vi "nanocal -- nuclear schottky fit -- 2x2 -- V9.vi"() -> ()   [LabVIEW 2021] (continued)
\"Imoff\" -> 0.000000000000   ,  \"στ1\" -> 0.008245172960   ,  \"στS\" -> 0.001836119711   ,  \"στN\" -> 0.000000000000    |>   , \n\"IDS0301_210831_RAW_cal__sam_\" ->   <|    \"ζ\" -> 0.050368719514   ,  \"τ1\" -> 0.024372679774   ,  \"τS\" -> 0.056652990002   ,  \"τN\" -> 0.018868210601   ,  \"τC\" -> 0.002169557672   ,  \"κ0\" -> 0.000000001890   ,  \"mm1\" -> 0.000100537132   ,  \"mm2\" -> 0.016885854065   ,  \"mm3\" -> 0.088880953022   ,  \"T\" -> 0.300000000000   ,  \"B\" -> 12.000000000000   ,  \"θ\" -> 30.000000000000   ,  \"Reoff\" -> -5240963.855421677230   ,  \"Imoff\" -> 0.000000000000   ,  \"στ1\" -> 0.000000000000   ,  \"στS\" -> 0.000000000000   ,  \"στN\" -> 0.000000000000    |>   , \n\"IDS0302_210831_RAW_cal__ref_\" ->   <|    \"ζ\" -> 0.118276511674   ,  \"τ1\" -> 0.024667236768   ,  \"τS\" -> 0.048709348590   ,  \"τN\" -> 0.031529020299   ,  \"τC\" -> 0.001279390112   ,  \"κ0\" -> 0.000000001362   ,  \"mm1\" -> 0.000132517053   ,  \"mm2\" -> 0.013437351030   ,  \"mm3\" -> 0.102105442061   ,  \"T\" -> 0.250000000000   ,  \"B\" -> 12.000000000000   ,  \"θ\" -> 30.000000000000   ,  \"Reoff\" -> -14030120.481927707800   ,  \"Imoff\" -> 0.000000000000   ,  \"στ1\" -> 0.005527591080   ,  \"στS\" -> 0.002366766012   ,  \"στN\" -> 0.000000000000    |>   , \n\"IDS0302_210831_RAW_cal__sam_\" ->   <|    \"ζ\" -> 0.070275268573   ,  \"τ1\" -> 0.028026457127   ,  \"τS\" -> 0.065297867120   ,  \"τN\" -> 0.040008645873   ,  \"τC\" -> 0.001817885465   ,  \"κ0\" -> 0.000000001504   ,  \"mm1\" -> 0.000116520135   ,  \"mm2\" -> 0.015851021970   ,  \"mm3\" -> 0.126583756963   ,  \"T\" -> 0.250000000000   ,  \"B\" -> 12.000000000000   ,  \"θ\" -> 30.000000000000   ,  \"Reoff\" -> -8554216.867469877010   ,  \"Imoff\" -> 0.000000000000   ,  \"στ1\" -> 0.000000000000   ,  \"στS\" -> 0.000000000000   ,  \"στN\" -> 0.000000000000    |>   , \n\"IDS0303_210831_RAW_cal__ref_\" ->   <|    \"ζ\" -> 0.210201005272   ,  \"τ1\" -> 0.036306230706   ,  \"τS\" -> 0.066320996268   ,  \"τN\" -> 0.080911010033   ,  \"τC\" -> 0.001077377701   ,  \"κ0\" -> 0.000000001046   ,  \"mm1\" -> 0.000185060428   ,  \"mm2\" -> 0.014681839337   ,  \"mm3\" -> 0.200697030676   ,  \"T\" -> 0.200000000000   ,  \"B\" -> 12.000000000000   ,  \"θ\" -> 30.000000000000   ,  \"Reoff\" -> -29165662.650602400300   ,  \"Imoff\" -> 0.000000000000   ,  \"στ1\" -> 0.007631270383   ,  \"στS\" -> 0.005042040043   ,  \"στN\" -> 0.000000000000    |>   , \n\"IDS0303_210831_RAW_cal__sam_\" ->   <|    \"ζ\" -> 0.127771364483   ,  \"τ1\" -> 0.034431916362   ,  \"τS\" -> 0.086066228156   ,  \"τN\" -> 0.103317216156   ,  \"τC\" -> 0.001469970272   ,  \"κ0\" -> 0.000000001169   ,  \"mm1\" -> 0.000164317810   ,  \"mm2\" -> 0.014420189715   ,  \"mm3\" -> 0.234898604511   ,  \"T\" -> 0.200000000000   ,  \"B\" -> 12.000000000000   ,  \"θ\" -> 30.000000000000   ,  \"Reoff\" -> -17831325.301204815500   ,  \"Imoff\" -> 0.000000000000   ,  \"στ1\" -> 0.000000000000   ,  \"στS\" -> 0.000000000000   ,  \"στN\" -> 0.000000000000    |>   , \n\"IDS0304_210831_RAW_cal__ref_\" ->   <|    \"ζ\" -> 0.269991588498   ,  \"τ1\" -> 0.042008612133   ,  \"τS\" -> 0.092789631538   ,  \"τN\" -> 0.170188261604   ,  \"τC\" -> 0.001076825929   ,  \"κ0\" -> 0.000000000745   ,  \"mm1\" -> 0.000227270912   ,  \"mm2\" -> 0.013732742400   ,  \"mm3\" -> 0.363105137001   ,  \"T\" -> 0.170000000000   ,  \"B\" -> 12.000000000000   ,  \"θ\" -> 30.000000000000   ,  \"Reoff\" -> -52171686.746987946300   ,  \"Imoff\" -> 0.000000000000   ,  \"στ1\" -> 0.010619336598   ,  \"στS\" -> 0.010896322396   ,  \"στN\" -> 0.000000000000    |>   , \n\"IDS0304_210831_RAW_cal__sam_\" ->   <|    \"ζ\" -> 0.166070461716   ,  \"τ1\" -> 0.041003941798   ,  \"τS\" -> 0.114733330952   ,  \"τN\" -> 0.164402286708   ,  \"τC\" -> 0.001371627013   ,  \"κ0\" -> 0.000000000890   ,  \"mm1\" -> 0.000193629021   ,  \"mm2\" -> 0.015725118152   ,  \"mm3\" -> 0.351948620204   ,  \"T\" -> 0.170000000000   ,  \"B\" -> 12.000000000000   ,  \"θ\" -> 30.000000000000   ,  \"Reoff\" -> -32409638.554216861700   ,  \"Imoff\" -> 0.000000000000   ,  \"στ1\" -> 0.000000000000   ,  \"στS\" -> 0.000000000000   ,  \"στN\" -> 0.000000000000    |>   , \n\"IDS0305_210831_RAW_cal__ref_\" ->   <|    \"ζ\" -> 0.281505704242   ,  \"τ1\" -> 0.044410384222   ,  \"τS\" -> 0.104666316175   ,  \"τN\" -> 0.238180601074   ,  \"τC\" -> 0.001077670144   ,  \"κ0\" -> 0.000000000630   ,  \"mm1\" -> 0.000235234007   ,  \"mm2\" -> 0.012702965231   ,  \"mm3\" -> 0.471910135265   ,  \"T\" -> 0.160000000000   ,  \"B\" -> 12.000000000000   ,  \"θ\" -> 30.000000000000   ,  \"Reoff\" -> -64885542.168674700000   ,  \"Imoff\" -> 0.000000000000   ,  \"στ1\" -> 0.013415612751   ,  \"στS\" -> 0.014884617591   ,  \"στN\" -> 0.000000000000    |>   , \n\"IDS0305_210831_RAW_cal__sam_\" ->   <|    \"ζ\" -> 0.168984978681   ,  \"τ1\" -> 0.042944879888   ,  \"τS\" -> 0.137797235983   ,  \"τN\" -> 0.201278537585   ,  \"τC\" -> 0.001423239236   ,  \"κ0\" -> 0.000000000771   ,  \"mm1\" -> 0.000204183123   ,  \"mm2\" -> 0.016435652766   ,  \"mm3\" -> 0.424102769171   ,  \"T\" -> 0.160000000000   ,  \"B\" -> 12.000000000000   ,  \"θ\" -> 30.000000000000   ,  \"Reoff\" -> -36385542.168674692500   ,  \"Imoff\" -> 0.000000000000   ,  \"στ1\" -> 0.000000000000   ,  \"στS\" -> 0.000000000000   ,  \"στN\" -> 0.000000000000    |>   , \n\"IDS0306_210831_RAW_cal__ref_\" ->   <|    \"ζ\" -> 0.013593052641   ,  \"τ1\" -> 0.010989385662   ,  \"τS\" -> 0.007947176041   ,  \"τN\" -> 0.000037757079   ,  \"τC\" -> 0.003572854733   ,  \"κ0\" -> 0.000000023548   ,  \"mm1\" -> 0.000033287498   ,  \"mm2\" -> 0.010587625602   ,  \"mm3\" -> 0.012034800032   ,  \"T\" -> 3.100000000000   ,  \"B\" -> 12.000000000000   ,  \"θ\" -> 30.000000000000   ,  \"Reoff\" -> 0.000000000000   ,  \"Imoff\" -> 0.000000000000   ,  \"στ1\" -> 0.000000000000   ,  \"στS\" -> 0.000000000000   ,  \"στN\" -> 0.000000000000    |>   , \n\"IDS0306_210831_RAW_cal__sam_\" ->   <|    \"ζ\" -> 0.007685785961   ,  \"τ1\" -> 0.018036205476   ,  \"τS\" -> 0.008821186550   ,  \"τN\" -> 0.000090733660   ,  \"τC\" -> 0.005794291982   ,  \"κ0\" -> 0.000000024405   ,  \"mm1\" -> 0.000026803010   ,  \"mm2\" -> 0.014306219949   ,  \"mm3\" -> 0.018477889820   ,  \"T\" -> 3.100000000000   ,  \"B\" -> 12.000000000000   ,  \"θ\" -> 30.000000000000   ,  \"Reoff\" -> -62000.000000000000   ,  \"Imoff\" -> 0.000000000000   ,  \"στ1\" -> 0.000000000000   ,  \"στS\" -> 0.000000000000   ,  \"στN\" -> 0.000000000000    |>   , \n\"IDS0310_210901_RAW_cal__ref_\" ->   <|    \"ζ\" -> 0.294196069585   ,  \"τ1\" -> 0.054258754823   ,  \"τS\" -> 0.066187792705   ,  \"τN\" -> 0.210307390595   ,  \"τC\" -> 0.001028009628   ,  \"κ0\" -> 0.000000000624   ,  \"mm1\" -> 0.000231504342   ,  \"mm2\" -> 0.011693954387   ,  \"mm3\" -> 0.401200285208   ,  \"T\" -> 0.157000000000   ,  \"B\" -> 12.000000000000   ,  \"θ\" -> 45.000000000000   ,  \"Reoff\" -> -66590361.445783138300   ,  \"Imoff\" -> 0.000000000000   ,  \"στ1\" -> 0.021984252892   ,  \"στS\" -> 0.027799498625   ,  \"στN\" -> 0.000000000000    |>   , \n\"IDS0310_210901_RAW_cal__sam_\" ->   <|    \"ζ\" -> 0.295520923520   ,  \"τ1\" -> 0.054772440405   ,  \"τS\" -> 0.071814005451   ,  \"τN\" -> 0.249593767169   ,  \"τC\" -> 0.001103632155   ,  \"κ0\" -> 0.000000000625   ,  \"mm1\" -> 0.000249422174   ,  \"mm2\" -> 0.011160480416   ,  \"mm3\" -> 0.460856664381   ,  \"T\" -> 0.157000000000   ,  \"B\" -> 12.000000000000   ,  \"θ\" -> 45.000000000000   ,  \"Reoff\" -> 0.000000000000   ,  \"Imoff\" -> 0.000000000000   ,  \"στ1\" -> 0.000000000000   ,  \"στS\" -> 0.000000000000   ,  \"στN\" -> 0.000000000000    |>   , \n\"IDS0311_210901_RAW_cal__ref_\" ->   <|    \"ζ\" -> 0.508858563878   ,  \"τ1\" -> 0.072484057695   ,  \"τS\" -> 0.091005153910   ,  \"τN\" -> 0.493200178379   ,  \"τC\" -> 0.000985068264   ,  \"κ0\" -> 0.000000000428   ,  \"mm1\" -> 0.000330595844   ,  \"mm2\" -> 0.010594734788   ,  \"mm3\" -> 0.944027014014   ,  \"T\" -> 0.120000000000   ,  \"B\" -> 12.000000000000   ,  \"θ\" -> 45.000000000000   ,  \"Reoff\" -> -111015060.240963846000   ,  \"Imoff\" -> 0.000000000000   ,  \"στ1\" -> 0.030760368517   ,  \"στS\" -> 0.002434782882   ,  \"στN\" -> 0.000000000000    |>   , \n\"IDS0311_210901_RAW_cal__sam_\" ->   <|    \"ζ\" -> 0.523545279740   ,  \"τ1\" -> 0.065613539167   ,  \"τS\" -> 0.100000000000   ,  \"τN\" -> 0.424083114177   ,  \"τC\" -> 0.000911255863   ,  \"κ0\" -> 0.000000000418   ,  \"mm1\" -> 0.000311888140   ,  \"mm2\" -> 0.011767552098   ,  \"mm3\" -> 0.852909709588   ,  \"T\" -> 0.120000000000   ,  \"B\" -> 12.000000000000   ,  \"θ\" -> 45.000000000000   ,  \"Reoff\" -> 0.000000000000   ,  \"Imoff\" -> 0.000000000000   ,  \"στ1\" -> 0.000000000000   ,  \"στS\" -> 0.000000000000   ,  \"στN\" -> 0.000000000000    |>   , \n\"IDS0312_210901_RAW_cal__ref_\" ->   <|    \"ζ\" -> 0.259527657087   ,  \"τ1\" -> 0.050950801212   ,  \"τS\" -> 0.056257064354   ,  \"τN\" -> 0.162412214705   ,  \"τC\" -> 0.001029454962   ,  \"κ0\" -> 0.000000000750   ,  \"mm1\" -> 0.000209665786   ,  \"mm2\" -> 0.011572567257   ,  \"mm3\" -> 0.315618027862   ,  \"T\" -> 0.170000000000   ,  \"B\" -> 12.000000000000   ,  \"θ\" -> 45.000000000000   ,  \"Reoff\" -> -47551204.819277107700   ,  \"Imoff\" -> 0.000000000000   ,  \"στ1\" -> 0.007568346917   ,  \"στS\" -> 0.006727038440   ,  \"στN\" -> 0.000000000000    |>   , \n\"IDS0312_210901_RAW_cal__sam_\" ->   <|    \"ζ\" -> 0.273742116471   ,  \"τ1\" -> 0.052262909995   ,  \"τS\" -> 0.060554036646   ,  \"τN\" -> 0.154269705680   ,  \"τC\" -> 0.001074144337   ,  \"κ0\" -> 0.000000000753   ,  \"mm1\" -> 0.000228314156   ,  \"mm2\" -> 0.012990527394   ,  \"mm3\" -> 0.313748261000   ,  \"T\" -> 0.170000000000   ,  \"B\" -> 12.000000000000   ,  \"θ\" -> 45.000000000000   ,  \"Reoff\" -> 0.000000000000   ,  \"Imoff\" -> 0.000000000000   ,  \"στ1\" -> 0.000000000000   ,  \"στS\" -> 0.000000000000   ,  \"στN\" -> 0.000000000000    |>   , \n\"IDS0313_210901_RAW_cal__ref_\" ->   <|    \"ζ\" -> 0.214632480491   ,  \"τ1\" -> 0.045379665546   ,  \"τS\" -> 0.046142273352   ,  \"τN\" -> 0.090406420650   ,  \"τC\" -> 0.001068824468   ,  \"κ0\" -> 0.000000001040   ,  \"mm1\" -> 0.000185914799   ,  \"mm2\" -> 0.012974151189   ,  \"mm3\" -> 0.199144902930   ,  \"T\" -> 0.200000000000   ,  \"B\" -> 12.000000000000   ,  \"θ\" -> 45.000000000000   ,  \"Reoff\" -> -30325301.204819276900   ,  \"Imoff\" -> 0.000000000000   ,  \"στ1\" -> 0.006255922124   ,  \"στS\" -> 0.003795789504   ,  \"στN\" -> 0.000000000000    |>   , \n\"IDS0313_210901_RAW_cal__sam_\" ->   <|    \"ζ\" -> 0.215688135788   ,  \"τ1\" -> 0.043710888546   ,  \"τS\" -> 0.044756474141   ,  \"τN\" -> 0.090222547904   ,  \"τC\" -> 0.001049781785   ,  \"κ0\" -> 0.000000001047   ,  \"mm1\" -> 0.000183308759   ,  \"mm2\" -> 0.012306282012   ,  \"mm3\" -> 0.196363475241   ,  \"T\" -> 0.200000000000   ,  \"B\" -> 12.000000000000   ,  \"θ\" -> 45.000000000000   ,  \"Reoff\" -> 0.000000000000   ,  \"Imoff\" -> 0.000000000000   ,  \"στ1\" -> 0.000000000000   ,  \"στS\" -> 0.000000000000   ,  \"στN\" -> 0.000000000000    |>   , \n\"IDS0314_210901_RAW_cal__ref_\" ->   <|    \"ζ\" -> 0.122092266901   ,  \"τ1\" -> 0.034197829393   ,  \"τS\" -> 0.036704742397   ,  \"τN\" -> 0.033844850691   ,  \"τC\" -> 0.001292192977   ,  \"κ0\" -> 0.000000001353   ,  \"mm1\" -> 0.000136749869   ,  \"mm2\" -> 0.014475424463   ,  \"mm3\" -> 0.100041000875   ,  \"T\" -> 0.255000000000   ,  \"B\" -> 12.000000000000   ,  \"θ\" -> 45.000000000000   ,  \"Reoff\" -> -14006024.096385538600   ,  \"Imoff\" -> 0.000000000000   ,  \"στ1\" -> 0.005419306546   ,  \"στS\" -> 0.001902499220   ,  \"στN\" -> 0.000000000000    |>   , \n\"IDS0314_210901_RAW_cal__sam_\" ->   <|    \"ζ\" -> 0.118583992968   ,  \"τ1\" -> 0.035232851003   ,  \"τS\" -> 0.037458022816   ,  \"τN\" -> 0.033724509363   ,  \"τC\" -> 0.001440922263   ,  \"κ0\" -> 0.000000001360   ,  \"mm1\" -> 0.000148167008   ,  \"mm2\" -> 0.015055022209   ,  \"mm3\" -> 0.101094225124   ,  \"T\" -> 0.255000000000   ,  \"B\" -> 12.000000000000   ,  \"θ\" -> 45.000000000000   ,  \"Reoff\" -> 0.000000000000   ,  \"Imoff\" -> 0.000000000000   ,  \"στ1\" -> 0.000000000000   ,  \"στS\" -> 0.000000000000   ,  \"στN\" -> 0.000000000000    |>   , \n\"IDS0315_210901_RAW_cal__ref_\" ->   <|    \"ζ\" -> 0.083764042578   ,  \"τ1\" -> 0.028404690940   ,  \"τS\" -> 0.032596022406   ,  \"τN\" -> 0.016694646015   ,  \"τC\" -> 0.001528847398   ,  \"κ0\" -> 0.000000001734   ,  \"mm1\" -> 0.000113603931   ,  \"mm2\" -> 0.015380769719   ,  \"mm3\" -> 0.067858618758   ,  \"T\" -> 0.300000000000   ,  \"B\" -> 12.000000000000   ,  \"θ\" -> 45.000000000000   ,  \"Reoff\" -> -7659638.554216861730   ,  \"Imoff\" -> 0.000000000000   ,  \"στ1\" -> 0.006630999900   ,  \"στS\" -> 0.001474626278   ,  \"στN\" -> 0.000000000000    |>   , \n\"IDS0315_210901_RAW_cal__sam_\" ->   <|    \"ζ\" -> 0.085152769414   ,  \"τ1\" -> 0.029001116263   ,  \"τS\" -> 0.032604663993   ,  \"τN\" -> 0.016878763935   ,  \"τC\" -> 0.001443524845   ,  \"κ0\" -> 0.000000001728   ,  \"mm1\" -> 0.000109149910   ,  \"mm2\" -> 0.015549242931   ,  \"mm3\" -> 0.068483327123   ,  \"T\" -> 0.300000000000   ,  \"B\" -> 12.000000000000   ,  \"θ\" -> 45.000000000000   ,  \"Reoff\" -> 0.000000000000   ,  \"Imoff\" -> 0.000000000000   ,  \"στ1\" -> 0.000000000000   ,  \"στS\" -> 0.000000000000   ,  \"στN\" -> 0.000000000000    |>   , \n\"IDS0316_210901_RAW_cal__ref_\" ->   <|    \"ζ\" -> 0.059431977734   ,  \"τ1\" -> 0.025344964439   ,  \"τS\" -> 0.030187831822   ,  \"τN\" -> 0.009997229668   ,  \"τC\" -> 0.001837989117   ,  \"κ0\" -> 0.000000002120   ,  \"mm1\" -> 0.000097780180   ,  \"mm2\" -> 0.015899559471   ,  \"mm3\" -> 0.053758953075   ,  \"T\" -> 0.360000000000   ,  \"B\" -> 12.000000000000   ,  \"θ\" -> 45.000000000000   ,  \"Reoff\" -> -3126506.024096369740   ,  \"Imoff\" -> 0.000000000000   ,  \"στ1\" -> 0.002854320609   ,  \"στS\" -> 0.000336853437   ,  \"στN\" -> 0.000497959558    |>   , \n\"IDS0316_210901_RAW_cal__sam_\" ->   <|    \"ζ\" -> 0.061011838044   ,  \"τ1\" -> 0.025440548989   ,  \"τS\" -> 0.030028053978   ,  \"τN\" -> 0.010140731955   ,  \"τC\" -> 0.001895079687   ,  \"κ0\" -> 0.000000002115   ,  \"mm1\" -> 0.000103163383   ,  \"mm2\" -> 0.015856737579   ,  \"mm3\" -> 0.053995285109   ,  \"T\" -> 0.360000000000   ,  \"B\" -> 12.000000000000   ,  \"θ\" -> 45.000000000000   ,  \"Reoff\" -> 0.000000000000   ,  \"Imoff\" -> 0.000000000000   ,  \"στ1\" -> 0.000000000000   ,  \"στS\" -> 0.000000000000   ,  \"στN\" -> 0.000000000000    |>   , \n\"IDS0317_210901_RAW_cal__ref_\" ->   <|    \"ζ\" -> 0.044144689760   ,  \"τ1\" -> 0.021030727933   ,  \"τS\" -> 0.027802850368   ,  \"τN\" -> 0.005306153044   ,  \"τC\" -> 0.002039269513   ,  \"κ0\" -> 0.000000002643   ,  \"mm1\" -> 0.000080764182   ,  \"mm2\" -> 0.015493151772   ,  \"mm3\" -> 0.042066671588   ,  \"T\" -> 0.430000000000   ,  \"B\" -> 12.000000000000   ,  \"θ\" -> 45.000000000000   ,  \"Reoff\" -> -2219879.518072277310   ,  \"Imoff\" -> 0.000000000000   ,  \"στ1\" -> 0.001811234684   ,  \"στS\" -> 0.000219110470   ,  \"στN\" -> 0.000329233021    |>   , \n\"IDS0317_210901_RAW_cal__sam_\" ->   <|    \"ζ\" -> 0.046686299518   ,  \"τ1\" -> 0.021011215626   ,  \"τS\" -> 0.027633142317   ,  \"τN\" -> 0.005348477555   ,  \"τC\" -> 0.002098477650   ,  \"κ0\" -> 0.000000002635   ,  \"mm1\" -> 0.000087510938   ,  \"mm2\" -> 0.015436995488   ,  \"mm3\" -> 0.042106596506   ,  \"T\" -> 0.430000000000   ,  \"B\" -> 12.000000000000   ,  \"θ\" -> 45.000000000000   ,  \"Reoff\" -> 0.000000000000   ,  \"Imoff\" -> 0.000000000000   ,  \"στ1\" -> 0.000000000000   ,  \"στS\" -> 0.000000000000   ,  \"στN\" -> 0.000000000000    |>   , \n\"IDS0318_210901_RAW_cal__ref_\" ->   <|    \"ζ\" -> 0.032848823108   ,  \"τ1\" -> 0.018119264501   ,  \"τS\" -> 0.025633128962   ,  \"τN\" -> 0.002741342485   ,  \"τC\" -> 0.002539258002   ,  \"κ0\" -> 0.000000003301   ,  \"mm1\" -> 0.000073876379   ,  \"mm2\" -> 0.015052062662   ,  \"mm3\" -> 0.034839122902   ,  \"T\" -> 0.530000000000   ,  \"B\" -> 12.000000000000   ,  \"θ\" -> 45.000000000000   ,  \"Reoff\" -> -1020408.163265287880   ,  \"Imoff\" -> 0.000000000000   ,  \"στ1\" -> 0.000541293278   ,  \"στS\" -> 0.000098746270   ,  \"στN\" -> 0.000060245222    |>   , \n\"IDS0318_210901_RAW_cal__sam_\" ->   <|    \"ζ\" -> 0.035204330012   ,  \"τ1\" -> 0.021011523093   ,  \"τS\" -> 0.025247316079   ,  \"τN\" -> 0.002718647875   ,  \"τC\" -> 0.003091727575   ,  \"κ0\" -> 0.000000003296   ,  \"mm1\" -> 0.000094318646   ,  \"mm2\" -> 0.017045496493   ,  \"mm3\" -> 0.035913922507   ,  \"T\" -> 0.530000000000   ,  \"B\" -> 12.000000000000   ,  \"θ\" -> 45.000000000000   ,  \"Reoff\" -> 0.000000000000   ,  \"Imoff\" -> 0.000000000000   ,  \"στ1\" -> 0.000000000000   ,  \"στS\" -> 0.000000000000   ,  \"στN\" -> 0.000000000000    |>   , \n\"IDS0319_210901_RAW_cal__ref_\" ->   <|    \"ζ\" -> 0.027000577828   ,  \"τ1\" -> 0.015965757563   ,  \"τS\" -> 0.024178947820   ,  \"τN\" -> 0.001643909719   ,  \"τC\" -> 0.002756663641   ,  \"κ0\" -> 0.000000003916   ,  \"mm1\" -> 0.000065386105   ,  \"mm2\" -> 0.014174024052   ,  \"mm3\" -> 0.031003100660   ,  \"T\" -> 0.620000000000   ,  \"B\" -> 12.000000000000   ,  \"θ\" -> 45.000000000000   ,  \"Reoff\" -> -897959.183673471211   ,  \"Imoff\" -> 0.000000000000   ,  \"στ1\" -> 0.001366735368   ,  \"στS\" -> 0.000249386446   ,  \"στN\" -> 0.000075862770    |>   , \n\"IDS0319_210901_RAW_cal__sam_\" ->   <|    \"ζ\" -> 0.030862035723   ,  \"τ1\" -> 0.019328530751   ,  \"τS\" -> 0.023568572597   ,  \"τN\" -> 0.001701966614   ,  \"τC\" -> 0.003453790534   ,  \"κ0\" -> 0.000000003906   ,  \"mm1\" -> 0.000090824021   ,  \"mm2\" -> 0.016669294779   ,  \"mm3\" -> 0.032072641980   ,  \"T\" -> 0.620000000000   ,  \"B\" -> 12.000000000000   ,  \"θ\" -> 45.000000000000   ,  \"Reoff\" -> 0.000000000000   ,  \"Imoff\" -> 0.000000000000   ,  \"στ1\" -> 0.000000000000   ,  \"στS\" -> 0.000000000000   ,  \"στN\" -> 0.000000000000    |>   , \n\"IDS0320_210901_RAW_cal__ref_\" ->   <|    \"ζ\" -> 0.020582548855   ,  \"τ1\" -> 0.014453445820   ,  \"τS\" -> 0.020307523387   ,  \"τN\" -> 0.000603631080   ,  \"τC\" -> 0.003979837118   ,  \"κ0\" -> 0.000000005461   ,  \"mm1\" -> 0.000067516424   ,  \"mm2\" -> 0.013684499465   ,  \"mm3\" -> 0.026022826375   ,  \"T\" -> 0.830000000000   ,  \"B\" -> 12.000000000000   ,  \"θ\" -> 45.000000000000   ,  \"Reoff\" -> -285714.285714287310   ,  \"Imoff\" -> 0.000000000000   ,  \"στ1\" -> 0.000994587731   ,  \"στS\" -> 0.000123451502   ,  \"στN\" -> 0.000021982366    |>   , \n\"IDS0320_210901_RAW_cal__sam_\" ->   <|    \"ζ\" -> 0.023591124045   ,  \"τ1\" -> 0.014910006225   ,  \"τS\" -> 0.019342950404   ,  \"τN\" -> 0.000752972387   ,  \"τC\" -> 0.004900413232   ,  \"κ0\" -> 0.000000005453   ,  \"mm1\" -> 0.000090864236   ,  \"mm2\" -> 0.013909604856   ,  \"mm3\" -> 0.026379958563   ,  \"T\" -> 0.830000000000   ,  \"B\" -> 12.000000000000   ,  \"θ\" -> 45.000000000000   ,  \"Reoff\" -> 0.000000000000   ,  \"Imoff\" -> 0.000000000000   ,  \"στ1\" -> 0.000000000000   ,  \"στS\" -> 0.000000000000   ,  \"στN\" -> 0.000000000000    |>   , \n\"IDS0321_210901_RAW_cal__ref_\" ->   <|    \"ζ\" -> 0.020614746765   ,  \"τ1\" -> 0.013682065369   ,  \"τS\" -> 0.016105139108   ,  \"τN\" -> 0.000397734649   ,  \"τC\" -> 0.005005824303   ,  \"κ0\" -> 0.000000007592   ,  \"mm1\" -> 0.000077785268   ,  \"mm2\" -> 0.013046561126   ,  \"mm3\" -> 0.022406619598   ,  \"T\" -> 1.130000000000   ,  \"B\" -> 12.000000000000   ,  \"θ\" -> 45.000000000000   ,  \"Reoff\" -> 0.000000000000   ,  \"Imoff\" -> 0.000000000000   ,  \"στ1\" -> 0.000000000000   ,  \"στS\" -> 0.000000000000   ,  \"στN\" -> 0.000000000000    |>   , \n\"IDS0321_210901_RAW_cal__sam_\" ->   <|    \"ζ\" -> 0.020215154826   ,  \"τ1\" -> 0.014105227254   ,  \"τS\" -> 0.015660924043   ,  \"τN\" -> 0.000525137036   ,  \"τC\" -> 0.005447728357   ,  \"κ0\" -> 0.000000007594   ,  \"mm1\" -> 0.000080798630   ,  \"mm2\" -> 0.013233003317   ,  \"mm3\" -> 0.022752418474   ,  \"T\" -> 1.130000000000   ,  \"B\" -> 12.000000000000   ,  \"θ\" -> 45.000000000000   ,  \"Reoff\" -> 0.000000000000   ,  \"Imoff\" -> 0.000000000000   ,  \"στ1\" -> 0.000000000000   ,  \"στS\" -> 0.000000000000   ,  \"στN\" -> 0.000000000000    |>   , \n\"IDS0322_210901_RAW_cal__ref_\" ->   <|    \"ζ\" -> 0.019557893298   ,  \"τ1\" -> 0.012446212333   ,  \"τS\" -> 0.011139553358   ,  \"τN\" -> 0.000114229396   ,  \"τC\" -> 0.005115315079   ,  \"κ0\" -> 0.000000013115   ,  \"mm1\" -> 0.000067933462   ,  \"mm2\" -> 0.012117833487   ,  \"mm3\" -> 0.016849643499   ,  \"T\" -> 1.900000000000   ,  \"B\" -> 12.000000000000   ,  \"θ\" -> 45.000000000000   ,  \"Reoff\" -> 0.000000000000   ,  \"Imoff\" -> 0.000000000000   ,  \"στ1\" -> 0.000000000000   ,  \"στS\" -> 0.000000000000   ,  \"στN\" -> 0.000000000000    |>   , \n\"IDS0322_210901_RAW_cal__sam_\" ->   <|    \"ζ\" -> 0.018090572724   ,  \"τ1\" -> 0.013314780956   ,  \"τS\" -> 0.010820835010   ,  \"τN\" -> 0.000265552167   ,  \"τC\" -> 0.005393540417   ,  \"κ0\" -> 0.000000013100   ,  \"mm1\" -> 0.000064590824   ,  \"mm2\" -> 0.012452255889   ,  \"mm3\" -> 0.017478420931   ,  \"T\" -> 1.900000000000   ,  \"B\" -> 12.000000000000   ,  \"θ\" -> 45.000000000000   ,  \"Reoff\" -> 0.000000000000   ,  \"Imoff\" -> 0.000000000000   ,  \"στ1\" -> 0.000000000000   ,  \"στS\" -> 0.000000000000   ,  \"στN\" -> 0.000000000000    |>   , \n\"IDS0323_210901_RAW_cal__ref_\" ->   <|    \"ζ\" -> 0.018290634783   ,  \"τ1\" -> 0.011707989393   ,  \"τS\" -> 0.007391181448   ,  \"τN\" -> 0.000042685582   ,  \"τC\" -> 0.004638632451   ,  \"κ0\" -> 0.000000023525   ,  \"mm1\" -> 0.000051768819   ,  \"mm2\" -> 0.011185443963   ,  \"mm3\" -> 0.012679246238   ,  \"T\" -> 3.100000000000   ,  \"B\" -> 12.000000000000   ,  \"θ\" -> 45.000000000000   ,  \"Reoff\" -> 0.000000000000   ,  \"Imoff\" -> 0.000000000000   ,  \"στ1\" -> 0.000000000000   ,  \"στS\" -> 0.000000000000   ,  \"στN\" -> 0.000000000000    |>   , \n\"IDS0323_210901_RAW_cal__sam_\" ->   <|    \"ζ\" -> 0.019438138135   ,  \"τ1\" -> 0.013521019406   ,  \"τS\" -> 0.007253169401   ,  \"τN\" -> 0.000154824830   ,  \"τC\" -> 0.004746579385   ,  \"κ0\" -> 0.000000023466   ,  \"mm1\" -> 0.000055371802   ,  \"mm2\" -> 0.011289401344   ,  \"mm3\" -> 0.014474817491   ,  \"T\" -> 3.100000000000   ,  \"B\" -> 12.000000000000   ,  \"θ\" -> 45.000000000000   ,  \"Reoff\" -> 0.000000000000   ,  \"Imoff\" -> 0.000000000000   ,  \"στ1\" -> 0.000000000000   ,  \"στS\" -> 0.000000000000   ,  \"στN\" -> 0.000000000000    |>   , \n\"IDS0324_210901_RAW_cal__ref_\" ->   <|    \"ζ\" -> 0.016342153608   ,  \"τ1\" -> 0.012470308436   ,  \"τS\" -> 0.004793459347   ,  \"τN\" -> 0.000012881713   ,  \"τC\" -> 0.003213848745   ,  \"κ0\" -> 0.000000058321   ,  \"mm1\" -> 0.000031257206   ,  \"mm2\" -> 0.008030763960   ,  \"mm3\" -> 0.012507023039   ,  \"T\" -> 5.700000000000   ,  \"B\" -> 12.000000000000   ,  \"θ\" -> 45.000000000000   ,  \"Reoff\" -> 0.000000000000   ,  \"Imoff\" -> 0.000000000000   ,  \"στ1\" -> 0.000000000000   ,  \"στS\" -> 0.000000000000   ,  \"στN\" -> 0.000000000000    |>   , \n\"IDS0324_210901_RAW_cal__sam_\" ->   <|    \"ζ\" -> 0.018573189054   ,  \"τ1\" -> 0.013304612245   ,  \"τS\" -> 0.003723860844   ,  \"τN\" -> 0.000084829442   ,  \"τC\" -> 0.004309703632   ,  \"κ0\" -> 0.000000058362   ,  \"mm1\" -> 0.000036954445   ,  \"mm2\" -> 0.007938616076   ,  \"mm3\" -> 0.013518175167   ,  \"T\" -> 5.700000000000   ,  \"B\" -> 12.000000000000   ,  \"θ\" -> 45.000000000000   ,  \"Reoff\" -> 0.000000000000   ,  \"Imoff\" -> 0.000000000000   ,  \"στ1\" -> 0.000000000000   ,  \"στS\" -> 0.000000000000   ,  \"στN\" -> 0.000000000000    |>   , \n\"IDS0330_210901_RAW_cal__ref_\" ->   <|    \"ζ\" -> 0.000000000000   ,  \"τ1\" -> 0.000000000000   ,  \"τS\" -> 0.000000000000   ,  \"τN\" -> 0.000000000000   ,  \"τC\" -> 0.000000000000   ,  \"κ0\" -> 0.000000000000   ,  \"mm1\" -> 0.000000000000   ,  \"mm2\" -> 0.000000000000   ,  \"mm3\" -> 0.000000000000   ,  \"T\" -> 0.197000000000   ,  \"B\" -> 1.000000000000   ,  \"θ\" -> 90.000000000000   ,  \"Reoff\" -> 0.000000000000   ,  \"Imoff\" -> 0.000000000000   ,  \"στ1\" -> 0.000000000000   ,  \"στS\" -> 0.000000000000   ,  \"στN\" -> 0.000000000000    |>   , \n\"IDS0330_210901_RAW_cal__sam_\" ->   <|    \"ζ\" -> 0.000000000000   ,  \"τ1\" -> 0.000000000000   ,  \"τS\" -> 0.000000000000   ,  \"τN\" -> 0.000000000000   ,  \"τC\" -> 0.000000000000   ,  \"κ0\" -> 0.000000000000   ,  \"mm1\" -> 0.000000000000   ,  \"mm2\" -> 0.000000000000   ,  \"mm3\" -> 0.000000000000   ,  \"T\" -> 0.197000000000   ,  \"B\" -> 1.000000000000   ,  \"θ\" -> 90.000000000000   ,  \"Reoff\" -> 0.000000000000   ,  \"Imoff\" -> 0.000000000000   ,  \"στ1\" -> 0.000000000000   ,  \"στS\" -> 0.000000000000   ,  \"στN\" -> 0.000000000000    |>   , \n\"IDS0331_210901_RAW_cal__ref_\" ->   <|    \"ζ\" -> 0.000000000000   ,  \"τ1\" -> 0.000000000000   ,  \"τS\" -> 0.000000000000   ,  \"τN\" -> 0.000000000000   ,  \"τC\" -> 0.000000000000   ,  \"κ0\" -> 0.000000000000   ,  \"mm1\" -> 0.000000000000   ,  \"mm2\" -> 0.000000000000   ,  \"mm3\" -> 0.000000000000   ,  \"T\" -> 0.197000000000   ,  \"B\" -> 2.000000000000   ,  \"θ\" -> 90.000000000000   ,  \"Reoff\" -> 0.000000000000   ,  \"Imoff\" -> 0.000000000000   ,  \"στ1\" -> 0.000000000000   ,  \"στS\" -> 0.000000000000   ,  \"στN\" -> 0.000000000000    |>   , \n\"IDS0331_210901_RAW_cal__sam_\" ->   <|    \"ζ\" -> 0.000000000000   ,  \"τ1\" -> 0.000000000000   ,  \"τS\" -> 0.000000000000   ,  \"τN\" -> 0.000000000000   ,  \"τC\" -> 0.000000000000   ,  \"κ0\" -> 0.000000000000   ,  \"mm1\" -> 0.000000000000   ,  \"mm2\" -> 0.000000000000   ,  \"mm3\" -> 0.000000000000   ,  \"T\" -> 0.197000000000   ,  \"B\" -> 2.000000000000   ,  \"θ\" -> 90.000000000000   ,  \"Reoff\" -> 0.000000000000   ,  \"Imoff\" -> 0.000000000000   ,  \"στ1\" -> 0.000000000000   ,  \"στS\" -> 0.000000000000   ,  \"στN\" -> 0.000000000000    |>   , \n\"IDS0335_210904_RAW_cal__ref_\" ->   <|    \"ζ\" -> 0.206204028371   ,  \"τ1\" -> 0.030267809159   ,  \"τS\" -> 0.083699658284   ,  \"τN\" -> 0.011315524001   ,  \"τC\" -> 0.001118356963   ,  \"κ0\" -> 0.000000001029   ,  \"mm1\" -> 0.000189441796   ,  \"mm2\" -> 0.025670987536   ,  \"mm3\" -> 0.120133432419   ,  \"T\" -> 0.197000000000   ,  \"B\" -> 5.000000000000   ,  \"θ\" -> 90.000000000000   ,  \"Reoff\" -> -27794554.455445542900   ,  \"Imoff\" -> 0.000000000000   ,  \"στ1\" -> 0.030199688034   ,  \"στS\" -> 0.003526382549   ,  \"στN\" -> 0.000000000000    |>   , \n\"IDS0335_210904_RAW_cal__sam_\" ->   <|    \"ζ\" -> 0.127476550533   ,  \"τ1\" -> 0.026692349363   ,  \"τS\" -> 0.111739634553   ,  \"τN\" -> 0.012149249884   ,  \"τC\" -> 0.001469649387   ,  \"κ0\" -> 0.000000001130   ,  \"mm1\" -> 0.000164458900   ,  \"mm2\" -> 0.023578369229   ,  \"mm3\" -> 0.144100982695   ,  \"T\" -> 0.197000000000   ,  \"B\" -> 5.000000000000   ,  \"θ\" -> 90.000000000000   ,  \"Reoff\" -> -19117469.879518091700   ,  \"Imoff\" -> 0.000000000000   ,  \"στ1\" -> 0.000000000000   ,  \"στS\" -> 0.000000000000   ,  \"στN\" -> 0.000000000000    |>   , \n\"IDS0336_210904_RAW_cal__ref_\" ->   <|    \"ζ\" -> 0.369061948092   ,  \"τ1\" -> 0.041711176697   ,  \"τS\" -> 0.225950048302   ,  \"τN\" -> 0.066003099748   ,  \"τC\" -> 0.001407606072   ,  \"κ0\" -> 0.000000000381   ,  \"mm1\" -> 0.000378190489   ,  \"mm2\" -> 0.031503380077   ,  \"mm3\" -> 0.410939157824   ,  \"T\" -> 0.122000000000   ,  \"B\" -> 5.000000000000   ,  \"θ\" -> 90.000000000000   ,  \"Reoff\" -> -46126237.623762376600   ,  \"Imoff\" -> 0.000000000000   ,  \"στ1\" -> 0.041981174011   ,  \"στS\" -> 0.019738908124   ,  \"στN\" -> 0.000000000000    |>   , \n\"IDS0336_210904_RAW_cal__sam_\" ->   <|    \"ζ\" -> 0.192483765517   ,  \"τ1\" -> 0.038218926206   ,  \"τS\" -> 0.302700165376   ,  \"τN\" -> 0.092288910100   ,  \"τC\" -> 0.001788727736   ,  \"κ0\" -> 0.000000000500   ,  \"mm1\" -> 0.000287527431   ,  \"mm2\" -> 0.028741269140   ,  \"mm3\" -> 0.481996917433   ,  \"T\" -> 0.122000000000   ,  \"B\" -> 5.000000000000   ,  \"θ\" -> 90.000000000000   ,  \"Reoff\" -> 0.000000000000   ,  \"Imoff\" -> 0.000000000000   ,  \"στ1\" -> 0.000000000000   ,  \"στS\" -> 0.000000000000   ,  \"στN\" -> 0.000000000000    |>   , \n\"IDS0337_210904_RAW_cal__ref_\" ->   <|    \"ζ\" -> 0.291494561804   ,  \"τ1\" -> 0.036667876547   ,  \"τS\" -> 0.128215599927   ,  \"τN\" -> 0.021540574973   ,  \"τC\" -> 0.001127155281   ,  \"κ0\" -> 0.000000000640   ,  \"mm1\" -> 0.000253065243   ,  \"mm2\" -> 0.030442060863   ,  \"mm3\" -> 0.200509191202   ,  \"T\" -> 0.157000000000   ,  \"B\" -> 5.000000000000   ,  \"θ\" -> 90.000000000000   ,  \"Reoff\" -> -62465346.534653462500   ,  \"Imoff\" -> 0.000000000000   ,  \"στ1\" -> 0.039211636627   ,  \"στS\" -> 0.006414125500   ,  \"στN\" -> 0.000000000000    |>   , \n\"IDS0337_210904_RAW_cal__sam_\" ->   <|    \"ζ\" -> 0.174989526301   ,  \"τ1\" -> 0.032277116931   ,  \"τS\" -> 0.156061636315   ,  \"τN\" -> 0.033861256896   ,  \"τC\" -> 0.001461638306   ,  \"κ0\" -> 0.000000000742   ,  \"mm1\" -> 0.000216209109   ,  \"mm2\" -> 0.025810900049   ,  \"mm3\" -> 0.230869056407   ,  \"T\" -> 0.157000000000   ,  \"B\" -> 5.000000000000   ,  \"θ\" -> 90.000000000000   ,  \"Reoff\" -> -41753012.048192769300   ,  \"Imoff\" -> 0.000000000000   ,  \"στ1\" -> 0.000000000000   ,  \"στS\" -> 0.000000000000   ,  \"στN\" -> 0.000000000000    |>   , \n\"IDS0338_210904_RAW_cal__ref_\" ->   <|    \"ζ\" -> 0.269633076560   ,  \"τ1\" -> 0.032794135380   ,  \"τS\" -> 0.108453011647   ,  \"τN\" -> 0.017260666597   ,  \"τC\" -> 0.001066919164   ,  \"κ0\" -> 0.000000000733   ,  \"mm1\" -> 0.000225204386   ,  \"mm2\" -> 0.027393186252   ,  \"mm3\" -> 0.165852907980   ,  \"T\" -> 0.170000000000   ,  \"B\" -> 5.000000000000   ,  \"θ\" -> 90.000000000000   ,  \"Reoff\" -> -53299504.950495049400   ,  \"Imoff\" -> 0.000000000000   ,  \"στ1\" -> 0.032867428442   ,  \"στS\" -> 0.004982833917   ,  \"στN\" -> 0.000000000000    |>   , \n\"IDS0338_210904_RAW_cal__sam_\" ->   <|    \"ζ\" -> 0.165649151389   ,  \"τ1\" -> 0.028874600848   ,  \"τS\" -> 0.141983523605   ,  \"τN\" -> 0.021766467668   ,  \"τC\" -> 0.001383503895   ,  \"κ0\" -> 0.000000000838   ,  \"mm1\" -> 0.000195205233   ,  \"mm2\" -> 0.024502619119   ,  \"mm3\" -> 0.196435318758   ,  \"T\" -> 0.170000000000   ,  \"B\" -> 5.000000000000   ,  \"θ\" -> 90.000000000000   ,  \"Reoff\" -> -35397590.361445784600   ,  \"Imoff\" -> 0.000000000000   ,  \"στ1\" -> 0.000000000000   ,  \"στS\" -> 0.000000000000   ,  \"στN\" -> 0.000000000000    |>   , \n\"IDS0339_210904_RAW_cal__ref_\" ->   <|    \"ζ\" -> 0.118223949911   ,  \"τ1\" -> 0.026953810816   ,  \"τS\" -> 0.059687464570   ,  \"τN\" -> 0.005813068847   ,  \"τC\" -> 0.001318135171   ,  \"κ0\" -> 0.000000001341   ,  \"mm1\" -> 0.000136934905   ,  \"mm2\" -> 0.023512775569   ,  \"mm3\" -> 0.077866500712   ,  \"T\" -> 0.255000000000   ,  \"B\" -> 5.000000000000   ,  \"θ\" -> 90.000000000000   ,  \"Reoff\" -> -14245049.504950493600   ,  \"Imoff\" -> 0.000000000000   ,  \"στ1\" -> 0.036632926849   ,  \"στS\" -> 0.002605706336   ,  \"στN\" -> 0.000000000000    |>   , \n\"IDS0339_210904_RAW_cal__sam_\" ->   <|    \"ζ\" -> 0.070510248751   ,  \"τ1\" -> 0.022152847239   ,  \"τS\" -> 0.078660981887   ,  \"τN\" -> 0.006346817462   ,  \"τC\" -> 0.001852903257   ,  \"κ0\" -> 0.000000001477   ,  \"mm1\" -> 0.000119580835   ,  \"mm2\" -> 0.020081415868   ,  \"mm3\" -> 0.094806474219   ,  \"T\" -> 0.255000000000   ,  \"B\" -> 5.000000000000   ,  \"θ\" -> 90.000000000000   ,  \"Reoff\" -> -9000000.000000000000   ,  \"Imoff\" -> 0.000000000000   ,  \"στ1\" -> 0.000000000000   ,  \"στS\" -> 0.000000000000   ,  \"στN\" -> 0.000000000000    |>   , \n\"IDS0340_210904_RAW_cal__ref_\" ->   <|    \"ζ\" -> 0.082410022210   ,  \"τ1\" -> 0.025302969896   ,  \"τS\" -> 0.049616733190   ,  \"τN\" -> 0.002823484973   ,  \"τC\" -> 0.001541432070   ,  \"κ0\" -> 0.000000001718   ,  \"mm1\" -> 0.000114319399   ,  \"mm2\" -> 0.023099438171   ,  \"mm3\" -> 0.060392462102   ,  \"T\" -> 0.308000000000   ,  \"B\" -> 5.000000000000   ,  \"θ\" -> 90.000000000000   ,  \"Reoff\" -> -7868811.881188109520   ,  \"Imoff\" -> 0.000000000000   ,  \"στ1\" -> 0.036552733909   ,  \"στS\" -> 0.001615668069   ,  \"στN\" -> 0.000000000000    |>   , \n\"IDS0340_210904_RAW_cal__sam_\" ->   <|    \"ζ\" -> 0.049192434897   ,  \"τ1\" -> 0.021139048522   ,  \"τS\" -> 0.064524263818   ,  \"τN\" -> 0.003413094239   ,  \"τC\" -> 0.002227810965   ,  \"κ0\" -> 0.000000001879   ,  \"mm1\" -> 0.000101271202   ,  \"mm2\" -> 0.019728994700   ,  \"mm3\" -> 0.074815955705   ,  \"T\" -> 0.308000000000   ,  \"B\" -> 5.000000000000   ,  \"θ\" -> 90.000000000000   ,  \"Reoff\" -> -4933734.939759036530   ,  \"Imoff\" -> 0.000000000000   ,  \"στ1\" -> 0.000000000000   ,  \"στS\" -> 0.000000000000   ,  \"στN\" -> 0.000000000000    |>   , \n\"IDS0341_210904_RAW_cal__ref_\" ->   <|    \"ζ\" -> 0.059535652055   ,  \"τ1\" -> 0.024399428177   ,  \"τS\" -> 0.042628676419   ,  \"τN\" -> 0.001866665396   ,  \"τC\" -> 0.001976492813   ,  \"κ0\" -> 0.000000002092   ,  \"mm1\" -> 0.000106643977   ,  \"mm2\" -> 0.022574580065   ,  \"mm3\" -> 0.050839097951   ,  \"T\" -> 0.360000000000   ,  \"B\" -> 5.000000000000   ,  \"θ\" -> 90.000000000000   ,  \"Reoff\" -> -3485148.514851480720   ,  \"Imoff\" -> 0.000000000000   ,  \"στ1\" -> 0.049517186258   ,  \"στS\" -> 0.001491570893   ,  \"στN\" -> 0.000000000000    |>   , \n\"IDS0341_210904_RAW_cal__sam_\" ->   <|    \"ζ\" -> 0.036062522071   ,  \"τ1\" -> 0.018116162768   ,  \"τS\" -> 0.055032833309   ,  \"τN\" -> 0.002026723445   ,  \"τC\" -> 0.002755523522   ,  \"κ0\" -> 0.000000002282   ,  \"mm1\" -> 0.000091630452   ,  \"mm2\" -> 0.017261892165   ,  \"mm3\" -> 0.062635431951   ,  \"T\" -> 0.360000000000   ,  \"B\" -> 5.000000000000   ,  \"θ\" -> 90.000000000000   ,  \"Reoff\" -> -2587349.397590361540   ,  \"Imoff\" -> 0.000000000000   ,  \"στ1\" -> 0.000000000000   ,  \"στS\" -> 0.000000000000   ,  \"στN\" -> 0.000000000000    |>   , \n\"IDS0342_210904_RAW_cal__ref_\" ->   <|    \"ζ\" -> 0.044694741546   ,  \"τ1\" -> 0.020073823055   ,  \"τS\" -> 0.035925122531   ,  \"τN\" -> 0.001180968193   ,  \"τC\" -> 0.002238294537   ,  \"κ0\" -> 0.000000002627   ,  \"mm1\" -> 0.000090575996   ,  \"mm2\" -> 0.018946622284   ,  \"mm3\" -> 0.042039457171   ,  \"T\" -> 0.438000000000   ,  \"B\" -> 5.000000000000   ,  \"θ\" -> 90.000000000000   ,  \"Reoff\" -> -2688118.811881184580   ,  \"Imoff\" -> 0.000000000000   ,  \"στ1\" -> 0.000000000000   ,  \"στS\" -> 0.000039598396   ,  \"στN\" -> 0.000000000000    |>   , \n\"IDS0342_210904_RAW_cal__sam_\" ->   <|    \"ζ\" -> 0.027534849374   ,  \"τ1\" -> 0.019066527741   ,  \"τS\" -> 0.046236587360   ,  \"τN\" -> 0.001227722560   ,  \"τC\" -> 0.003332461518   ,  \"κ0\" -> 0.000000002852   ,  \"mm1\" -> 0.000083583563   ,  \"mm2\" -> 0.018352322518   ,  \"mm3\" -> 0.052734315722   ,  \"T\" -> 0.438000000000   ,  \"B\" -> 5.000000000000   ,  \"θ\" -> 90.000000000000   ,  \"Reoff\" -> -1846385.542168676850   ,  \"Imoff\" -> 0.000000000000   ,  \"στ1\" -> 0.000000000000   ,  \"στS\" -> 0.000000000000   ,  \"στN\" -> 0.000000000000    |>   , \n\"IDS0343_210904_RAW_cal__ref_\" ->   <|    \"ζ\" -> 0.035816355504   ,  \"τ1\" -> 0.018852618665   ,  \"τS\" -> 0.030539930714   ,  \"τN\" -> 0.000576682499   ,  \"τC\" -> 0.002754969701   ,  \"κ0\" -> 0.000000003271   ,  \"mm1\" -> 0.000087853298   ,  \"mm2\" -> 0.018179313354   ,  \"mm3\" -> 0.035571518608   ,  \"T\" -> 0.530000000000   ,  \"B\" -> 5.000000000000   ,  \"θ\" -> 90.000000000000   ,  \"Reoff\" -> -1891089.108910888430   ,  \"Imoff\" -> 0.000000000000   ,  \"στ1\" -> 0.000000000000   ,  \"στS\" -> 0.000000000000   ,  \"στN\" -> 0.000000000000    |>   , \n\"IDS0343_210904_RAW_cal__sam_\" ->   <|    \"ζ\" -> 0.023098882919   ,  \"τ1\" -> 0.017709986922   ,  \"τS\" -> 0.038881575014   ,  \"τN\" -> 0.000747654909   ,  \"τC\" -> 0.003803962289   ,  \"κ0\" -> 0.000000003538   ,  \"mm1\" -> 0.000078528513   ,  \"mm2\" -> 0.017209583260   ,  \"mm3\" -> 0.044770458303   ,  \"T\" -> 0.530000000000   ,  \"B\" -> 5.000000000000   ,  \"θ\" -> 90.000000000000   ,  \"Reoff\" -> -1599397.590361446140   ,  \"Imoff\" -> 0.000000000000   ,  \"στ1\" -> 0.000000000000   ,  \"στS\" -> 0.000000000000   ,  \"στN\" -> 0.000000000000    |>   , \n\"IDS0344_210904_RAW_cal__ref_\" ->   <|    \"ζ\" -> 0.030262302634   ,  \"τ1\" -> 0.017398280529   ,  \"τS\" -> 0.027078056707   ,  \"τN\" -> 0.000382363637   ,  \"τC\" -> 0.002680781698   ,  \"κ0\" -> 0.000000003878   ,  \"mm1\" -> 0.000072009464   ,  \"mm2\" -> 0.016908620237   ,  \"mm3\" -> 0.031389868421   ,  \"T\" -> 0.620000000000   ,  \"B\" -> 5.000000000000   ,  \"θ\" -> 90.000000000000   ,  \"Reoff\" -> -1891089.108910888430   ,  \"Imoff\" -> 0.000000000000   ,  \"στ1\" -> 0.000000000000   ,  \"στS\" -> 0.000000000000   ,  \"στN\" -> 0.000000000000    |>   , \n\"IDS0344_210904_RAW_cal__sam_\" ->   <|    \"ζ\" -> 0.019239644947   ,  \"τ1\" -> 0.016162010817   ,  \"τS\" -> 0.033688234899   ,  \"τN\" -> 0.000426792406   ,  \"τC\" -> 0.004393456024   ,  \"κ0\" -> 0.000000004224   ,  \"mm1\" -> 0.000073664779   ,  \"mm2\" -> 0.015859557336   ,  \"mm3\" -> 0.039393633044   ,  \"T\" -> 0.620000000000   ,  \"B\" -> 5.000000000000   ,  \"θ\" -> 90.000000000000   ,  \"Reoff\" -> -1105421.686746988450   ,  \"Imoff\" -> 0.000000000000   ,  \"στ1\" -> 0.000000000000   ,  \"στS\" -> 0.000000000000   ,  \"στN\" -> 0.000000000000    |>   , \n\"IDS0346_210904_RAW_cal__ref_\" ->   <|    \"ζ\" -> 0.358342122070   ,  \"τ1\" -> 0.051761802826   ,  \"τS\" -> 0.089859508524   ,  \"τN\" -> 0.270637714066   ,  \"τC\" -> 0.001160576368   ,  \"κ0\" -> 0.000000000399   ,  \"mm1\" -> 0.000303997839   ,  \"mm2\" -> 0.011999269265   ,  \"mm3\" -> 0.530297674424   ,  \"T\" -> 0.122000000000   ,  \"B\" -> 8.000000000000   ,  \"θ\" -> 90.000000000000   ,  \"Reoff\" -> -78405940.594059407700   ,  \"Imoff\" -> 0.000000000000   ,  \"στ1\" -> 0.018696549634   ,  \"στS\" -> 0.010329197801   ,  \"στN\" -> 0.000000000000    |>   , \n\"IDS0346_210904_RAW_cal__sam_\" ->   <|    \"ζ\" -> 0.199267253863   ,  \"τ1\" -> 0.050205114691   ,  \"τS\" -> 0.125855812683   ,  \"τN\" -> 0.296749666016   ,  \"τC\" -> 0.001624351903   ,  \"κ0\" -> 0.000000000535   ,  \"mm1\" -> 0.000267463038   ,  \"mm2\" -> 0.014047868056   ,  \"mm3\" -> 0.544331047407   ,  \"T\" -> 0.122000000000   ,  \"B\" -> 8.000000000000   ,  \"θ\" -> 90.000000000000   ,  \"Reoff\" -> -35716867.469879508000   ,  \"Imoff\" -> 0.000000000000   ,  \"στ1\" -> 0.000000000000   ,  \"στS\" -> 0.000000000000   ,  \"στN\" -> 0.000000000000    |>   , \n\"IDS0347_210906_RAW_cal__ref_\" ->   <|    \"ζ\" -> 0.284128861979   ,  \"τ1\" -> 0.040855237949   ,  \"τS\" -> 0.067239160062   ,  \"τN\" -> 0.100640688459   ,  \"τC\" -> 0.001094387721   ,  \"κ0\" -> 0.000000000641   ,  \"mm1\" -> 0.000239752131   ,  \"mm2\" -> 0.014685784170   ,  \"mm3\" -> 0.242603448199   ,  \"T\" -> 0.157000000000   ,  \"B\" -> 8.000000000000   ,  \"θ\" -> 90.000000000000   ,  \"Reoff\" -> -67247524.752475246800   ,  \"Imoff\" -> 0.000000000000   ,  \"στ1\" -> 0.009528946219   ,  \"στS\" -> 0.006641775518   ,  \"στN\" -> 0.000000000000    |>   , \n\"IDS0347_210906_RAW_cal__sam_\" ->   <|    \"ζ\" -> 0.169709128246   ,  \"τ1\" -> 0.042569783210   ,  \"τS\" -> 0.096466158196   ,  \"τN\" -> 0.116379310482   ,  \"τC\" -> 0.001498996005   ,  \"κ0\" -> 0.000000000766   ,  \"mm1\" -> 0.000215022431   ,  \"mm2\" -> 0.017656553883   ,  \"mm3\" -> 0.275164490520   ,  \"T\" -> 0.157000000000   ,  \"B\" -> 8.000000000000   ,  \"θ\" -> 90.000000000000   ,  \"Reoff\" -> -35716867.469879508000   ,  \"Imoff\" -> 0.000000000000   ,  \"στ1\" -> 0.000000000000   ,  \"στS\" -> 0.000000000000   ,  \"στN\" -> 0.000000000000    |>   , \n\"IDS0348_210906_RAW_cal__ref_\" ->   <|    \"ζ\" -> 0.229184446116   ,  \"τ1\" -> 0.036521753559   ,  \"τS\" -> 0.056643116422   ,  \"τN\" -> 0.063013769225 
